vi "Custom Filter.vi"(2 "dimension size":i32, 3 "Incremeter":i32, 4 "input":dbl format="%.2f") -> (0 "Filtered X":dbl[](array[numeric]), 1 "output":dbl format="%.2f")   [LabVIEW 2011]
uses:
  <vilib>/Analysis/NI_AALBase.lvlib
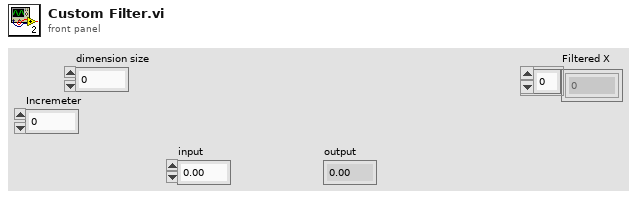
[diagram p1: front panel]
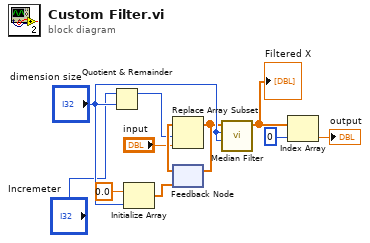
[diagram p0: block diagram]
diagram:
  n1 = Quotient & Remainder(x="Incremeter", y="dimension size") -> (x-y*floor(x/y)=w7:i32)  [unwired: 1 out]
  n2 = Initialize Array(0.0 ("element"), "dimension size") -> (w2:dbl[])
  n3 = feedback #1(w2) -> (w9:dbl[])
  n4 = Replace Array Subset(array=w9, new element="input", index=w7) -> (w8:dbl[])
  n5 = feedback-in #1(w8) -> ()
  n6 = call <vilib>:"Median Filter.vi"("right rank"="dimension size", "left rank"="dimension size", "X"=w8) -> ("Filtered X"=w4:dbl[])  [unwired: 7 in, 1 out]
  "Filtered X" <- w4
  n7 = Index Array(array=w4, index=0) -> (element=→"output":dbl)
